vi "Get Magnet.vi"(6 "Axis":T1, 8 "error in (no error)":errorcluster, 11 "instrument.PPMS":refnum<class "instrument.PPMS.lvclass">) -> (0 "error out":errorcluster, 1 "Status":string, 2 "B Field (T)":dbl, 3 "instrument.PPMS out":refnum<class "instrument.PPMS.lvclass">, 4 "Finished?":bool)   [LabVIEW 2019, in "instrument.PPMS.lvclass"]
uses:
  instrument.PPMS.lvclass
  Typedefs/PPMS.Magnet Status--cluster.ctl
  148e5cd9-bf63-4287-9255-410b676ea6b9.vi
  Typedefs/PPMS.Commands-enum.ctl
  C:/Program Files (x86)/National Instruments/LabVIEW 2019/user.lib/LevyLab/Levylab Instruments/Instrument Types/Cryostat/Instrument.Cryostat.lvclass
  C:/Program Files (x86)/National Instruments/LabVIEW 2019/user.lib/LevyLab/Levylab Instruments/SMOs/Instrument/Instrument.lvclass
  C:/Program Files (x86)/National Instruments/LabVIEW 2019/vi.lib/JKI/JKI SMO/SMO/SMO.lvclass
  <userlib>/LevyLab/Levylab Instruments/Instrument Types/Cryostat/Typedefs/Magnet Axis--Enum.ctl
  <userlib>/LevyLab/Levylab Instruments/Instrument Types/Cryostat/Instrument.Cryostat.lvclass
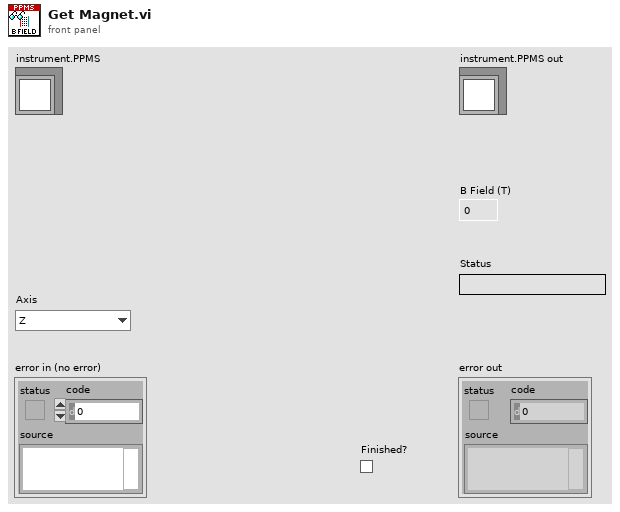
[diagram p1: front panel]
types:
  T1 = typedef "Instrument.Cryostat.lvclass/Magnet Axis--Enum.ctl" = enum16{"Z", "X", "Y"}
  T2 = typedef "instrument.PPMS.lvclass/PPMS.Commands-enum.ctl" = enum16{"Get Angle", "Get Helium Level", "Get Magnet", "Get Temperature", "Set Angle", "Set Chamber", "Set Magnet", "Set Temperature", "getAll"}
  T3 = typedef "instrument.PPMS.lvclass/PPMS.Magnet Status--cluster.ctl" = cluster{"Field (T)":dbl, "Magnet Status":string}
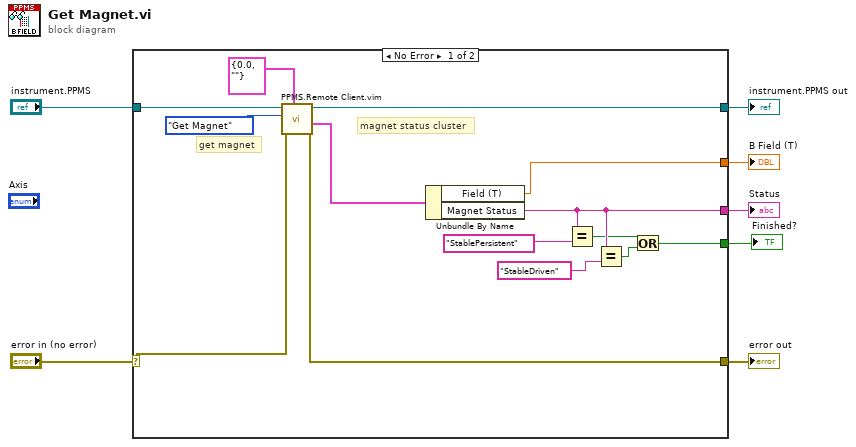
[diagram p0: block diagram]
diagram:
  n1 = case shown="No Error" "error in (no error)" {
    selector: "error in (no error)" -> [w12 w22]
    tunnel: [w11 w22] -> w7
    tunnel: [w13 w23] -> w6
    tunnel: "instrument.PPMS" -> [w21 w23]
    tunnel: [w20 _] -> w4
    tunnel: [w19 _] -> w3
    tunnel: [w18 _] -> w1
    frame No Error {
      # "magnet status cluster"
      # "get magnet"
      n2 = call "PPMS.Remote Client.vim"("Data Out type"=T3 {"Field (T)"=0.0, "Magnet Status"=""} ("input cluster"), "error in (no error)"=w12, "Command"=PPMS.Commands-enum."Get Magnet", "instrument.PPMS in"=w21) -> ("error out"=w11:errorcluster, "Data out"=w8:T3, "instrument.PPMS out"=w13:refnum<class "instrument.PPMS.lvclass">)  [unwired: 5 in]
      n3 = Unbundle By Name(w8) -> ("Field (T)"=w19:dbl, "Magnet Status"=w20:string)
      n4 = Equal?(x=w20, y="StablePersistent") -> (x = y?=w16:bool)
      n5 = Equal?(x=w20, y="StableDriven") -> (x = y?=w15:bool)
      n6 = Or(x=w16, y=w15) -> (x .or. y?=w18:bool)
    }
    frame Error {
    }
  }
  "error out" <- w7
  "instrument.PPMS out" <- w6
  "B Field (T)" <- w3
  "Status" <- w4
  "Finished?" <- w1
